vi "glsl_set_uniform_string.vi"(5 "Uniform Value":dbl[](array[numeric]), 6 "uniform index":i32, 7 "initial string":string) -> (3 "Uniform-setting string":string)   [LabVIEW 2019]
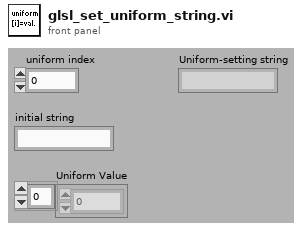
[diagram p1: front panel]
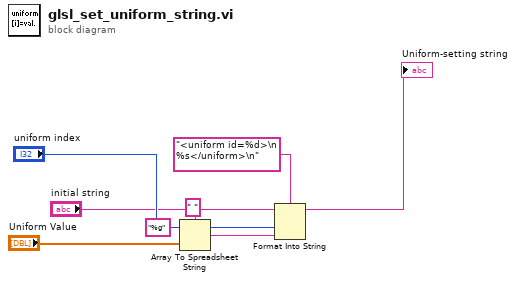
[diagram p0: block diagram]
diagram:
  n1 = Array To Spreadsheet String(delimiter (Tab)=" ", array="Uniform Value", 3:"%g" ("format string")) -> (spreadsheet string=w7:string)
  n2 = Format Into String(format string="<uniform id=%d>\n  %s</uniform>\n", initial string="initial string", "uniform index", w7) -> (resulting string=→"Uniform-setting string":string)  [unwired: 1 in, 1 out]
